vi "_logging_last_driver_VI.vi"(8 "error in":errorcluster caption="error in (no error)", 11 "Logging params in":variant) -> (0 "error out":errorcluster, 1 "VI changed":bool, 2 "New VI string":string, 3 "Logging params out":variant)   [LabVIEW 2020, in "Rohde&Schwarz RTx Oscilloscopes.lvlib" / "rsidr_core.lvlib"]
uses:
  rsidr_core.lvlib
  Match Regular Expression.xnode
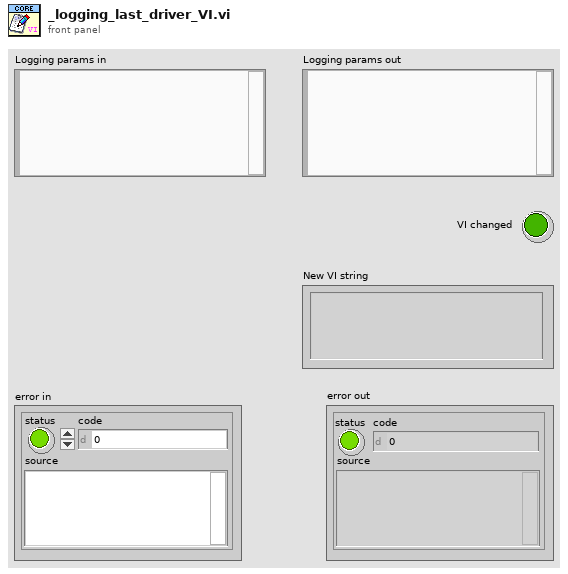
[diagram p1: front panel]
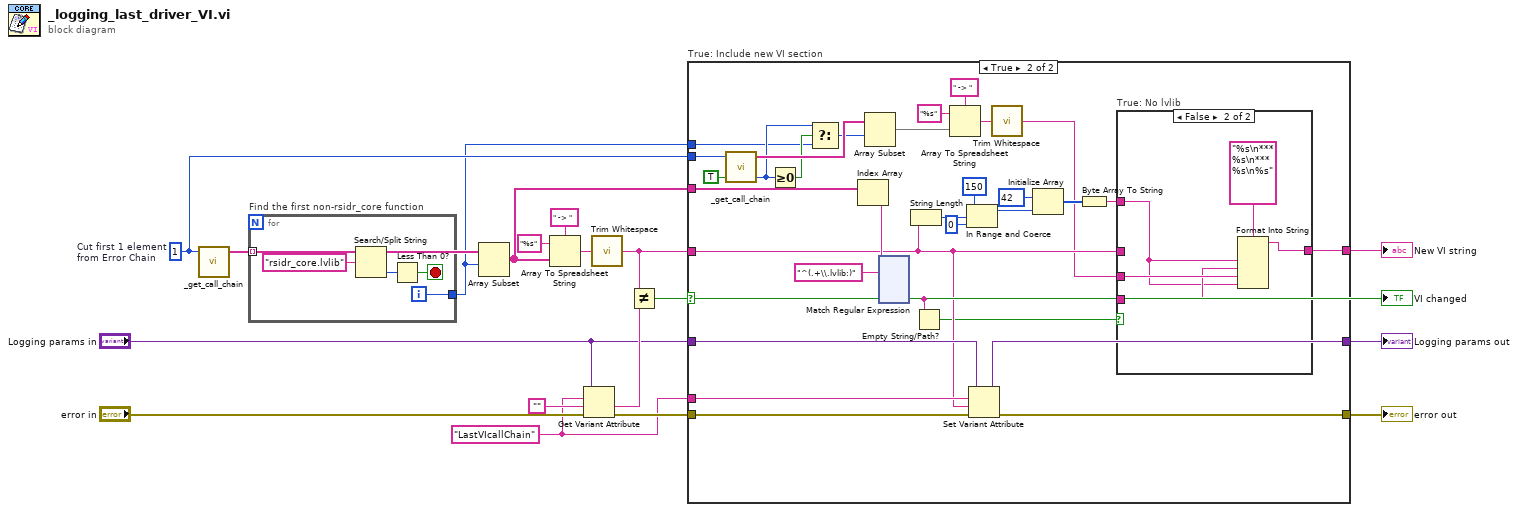
[diagram p0: block diagram]
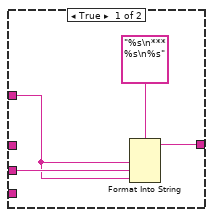
[diagram p3: hidden frame]
diagram:
  w3 = 1  # Cut first 1 element from Error Chain
  w6 = "LastVIcallChain" ("name")
  n1 = call "_get_call_chain.vi"("Cut first x elements\nfrom Error Chain (0)"=w3) -> ("Call chain out"=w12:string[])  [unwired: 2 in, 2 out]
  n2 = for "Find the first non-rsidr_core function" {
    tunnel: w12 -> [w21] mode=indexing
    tunnel: [w20] -> w1
    i -> [w20]
    stop <- w19 stop-if-true
    n3 = Search/Split String(string=w21, search string/char (-)="rsidr_core.lvlib" ("regular expression")) -> (offset of match=w22:i32)  [unwired: 1 in, 2 out]
    n4 = Less Than 0?(x=w22) -> (x < 0?=w19:bool)
  }
  n5 = Array Subset(array=w12, index=w1) -> (w2:string[])  [unwired: 1 in]
  n6 = Array To Spreadsheet String(delimiter (Tab)=" -> ", array=w2, 3:"%s" ("format string")) -> (spreadsheet string=w7:string)
  n7 = Get Variant Attribute(Variant="Logging params in", name=w6, default value (empty Variant)="" ("Empty String Constant"), error in="error in") -> (value=w17:string, error out=w15:errorcluster)  [unwired: 2 out]
  n8 = call "Trim Whitespace.vi"("string"=w7) -> ("trimmed string"=w5:string)  [unwired: 1 in]
  n9 = Not Equal?(x=w5, y=w17) -> (x != y?=w4:bool)
  "VI changed" <- w4
  n10 = case "True: Include new VI section" shown="True" w4 {
    tunnel: w15 -> [w24 w56]
    tunnel: "Logging params in" -> [w25 w55]
    tunnel: [w24 w54] -> w13
    tunnel: [w25 w53] -> w11
    tunnel: [_ w51] -> w10
    tunnel: w6 -> [_ w52]
    tunnel: w5 -> [_ w46]
    tunnel: w3 -> [_ w50]
    tunnel: w2 -> [_ w32]
    tunnel: w1 -> [_ w26]
    frame False {
    }
    frame True {
      n11 = call "_get_call_chain.vi"("Remove lvlib names (F)"=TRUE, "Cut first x elements\nfrom Error Chain (0)"=w50) -> ("ExVI index out"=w27:i32, "Call chain out"=w33:string[])  [unwired: 1 in, 1 out]
      n12 = Greater Or Equal To 0?(x=w27) -> (x >= 0?=w29:bool)
      n13 = Select(t=w27, s=w29, f=w26) -> (s? t:f=w28:i32)
      n14 = Index Array(array=w32) -> (element=w47:string)  [unwired: 1 in]
      n15 = Array Subset(array=w33, index=w28) -> (w31:string[])  [unwired: 1 in]
      n16 = xnode ("Match Regular Expression")("input string"=w47, "regular expression"="^(.+\\.lvlib:)" ("search string/char (-)")) -> ("submatch 1"=w37:string)  [unwired: 4 in, 5 out]
      n17 = String Length(string=w46) -> (length=w45:i32)
      n18 = Empty String/Path?(string/path=w37) -> (empty?=w38:bool)
      n19 = Array To Spreadsheet String(delimiter (Tab)=" -> ", array=w31, 3:"%s" ("format string")) -> (spreadsheet string=w34:string)
      n20 = In Range and Coerce(upper limit=150, x=w45, lower limit=0) -> (coerced(x)=w42:i32)  [unwired: 1 out]
      n21 = Set Variant Attribute(Variant=w55, name=w52, value=w46, error in=w56) -> (Variant out=w53:variant, error out=w54:errorcluster)  [unwired: 1 out]
      n22 = call "Trim Whitespace.vi"("string"=w34) -> ("trimmed string"=w30:string)  [unwired: 1 in]
      n23 = Initialize Array(u8 42 ("upper limit"), w42) -> (w40:u8[])
      n24 = Byte Array To String(unsigned byte array=w40) -> (string=w39:string)
      n25 = case "True: No lvlib" shown="False" w38 {
        tunnel: [w60 w65] -> w51
        tunnel: w46 -> [_ _]
        tunnel: w39 -> [w57 w61]
        tunnel: w37 -> [_ w62]
        tunnel: w30 -> [w58 w63]
        frame True {
          n26 = Format Into String(format string="%s\n***   %s\n%s", w57, w58, w57) -> (resulting string=w60:string)  [unwired: 2 in, 1 out]
        }
        frame False {
          n27 = Format Into String(format string="%s\n***   %s\n***   %s\n%s", w61, w62, w63, w61) -> (resulting string=w65:string)  [unwired: 2 in, 1 out]
        }
      }
    }
  }
  "error out" <- w13
  "Logging params out" <- w11
  "New VI string" <- w10
